vi "DSF.Engine.Framework.Tx.Async.vi"(8 "error in (no error)":errorcluster, 11 "Framework in":refnum<class "DSF.Engine.Framework.lvclass">) -> (0 "error out":errorcluster, 3 "Framework out":refnum<class "DSF.Engine.Framework.lvclass">)   [LabVIEW 2017, in "Data Sharing Framework Engine.lvlib" / "DSF.Engine.Framework.lvclass"]
uses:
  DSF.Engine.Framework.lvclass
  DSF.Engine.Framework.lvclass/DSF.Engine.Framework.ctl
  Plugin/DSF.Engine.Plugin.lvclass/DSF.Engine.Plugin.ctl
  Timing/DSF.Engine.Timing.lvclass/DSF.Engine.Timing.ctl
  Plugin/DSF.Engine.Plugin.Get Timing.vi
  Timing/DSF.Engine.Timing.Is Active Cycle.vi
  Timing/DSF.Engine.Timing.Get Decimation.vi
  Timing/DSF.Engine.Timing.Get Offset.vi
  Plugin/DSF.Engine.Plugin.lvclass
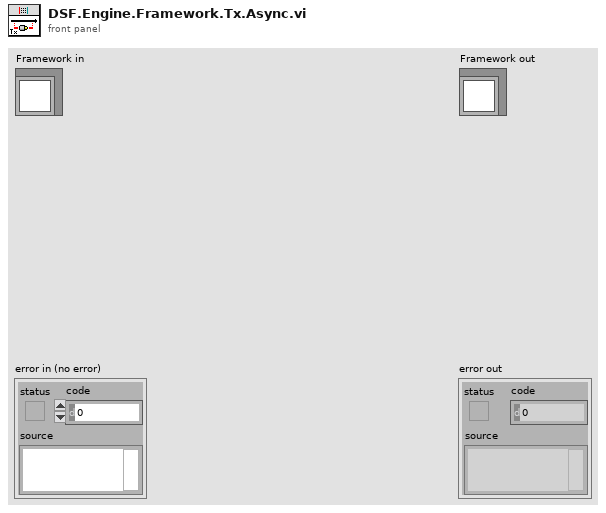
[diagram p1: front panel]
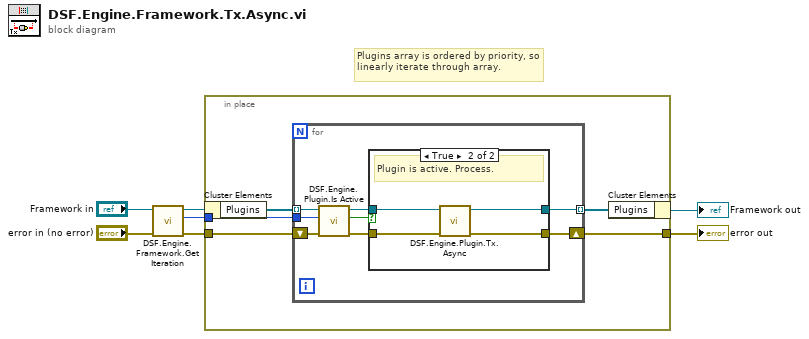
[diagram p0: block diagram]
diagram:
  # "Plugins array is ordered by priority, so linearly iterate through array."
  n1 = call "DSF.Engine.Framework.Get Iteration.vi"("Framework in"="Framework in") -> ("iteration"=w3:u64, "Framework out"=w1:refnum<class "DSF.Engine.Framework.lvclass">)  [unwired: 9 in]
  n2 = in-place {
    in-place-border: "error in (no error)" -> [w11]
    in-place-border: [w10] -> w5
    in-place-border: w3 -> [w7]
    n3 = in-place-cluster #1(w1) -> ("Plugins"=w9:refnum<class "DSF.Engine.Plugin.lvclass">[])
    n4 = for {
      tunnel: w9 -> [w15] mode=indexing
      tunnel: [w18] -> w8 mode=indexing
      shift-right: [w17] -> w10
      shift-left: w11 -> [w16]
      tunnel: w7 -> [w12]
      n5 = call "DSF.Engine.Plugin.Is Active.vi"("cycle count"=w12, "Plugin in"=w15) -> ("active this cycle?"=w13:bool, "Plugin out"=w14:refnum<class "DSF.Engine.Plugin.lvclass">)  [unwired: 8 in]
      n6 = case shown="True" w13 {
        tunnel: w14 -> [w20 w24]
        tunnel: [w20 w23] -> w18
        tunnel: [w19 w21] -> w17
        tunnel: w16 -> [w19 w22]
        frame False {
          # "Plugin is not active. Skip."
        }
        frame True {
          # "Plugin is active. Process."
          n7 = call "DSF.Engine.Plugin.Tx.Async.vi"("error in (no error)"=w22, "Plugin in"=w24) -> ("error out"=w21:errorcluster, "Plugin out"=w23:refnum<class "DSF.Engine.Plugin.lvclass">)  [unwired: 8 in]
        }
      }
    }
    n8 = in-place-cluster #1("Plugins"=w8) -> (→"Framework out":refnum<class "DSF.Engine.Framework.lvclass">)
  }
  "error out" <- w5
